vi "Actor Core.vi"(8 "error in":errorcluster, 11 "Test Node View in":refnum<class "Test Node View.lvclass">) -> (0 "error out":errorcluster, 3 "Actor out":refnum<class "Actor.lvclass">)   [LabVIEW 2013, in "Test Node View.lvlib" / "Test Node View.lvclass"]
doc: "(<B>Filename</B>: Actor Framework.lvlib:Actor.lvclass:Actor Core.vi)\n\nReceives messages to the actor, reacts to them, and initiates any error handling that may shut the actor down.\n\nDescendant classes may override this VI to append parallel tasks for the actor to complete while it handles messages. Overrides use the Call Parent Method node."
uses:
  Test Node View.lvclass
  <vilib>/ActorFramework/Actor/Actor.lvclass
  Resources/UI Controls/Tiles.ctl
  Resources/UI Controls/Tile.ctl
  Resources/UI Controls/Add Tile.ctl
  Resources/UI Controls/Delete Frame.ctl
  Test Node View.lvclass/Test Node View.ctl
  <vilib>/ActorFramework/Actor/Actor.lvclass/Actor.ctl
  <vilib>/ActorFrameworkMVC/View Actor/View Actor.lvclass
  <vilib>/ActorFramework/Message Enqueuer/Message Enqueuer.lvclass/Message Enqueuer.ctl
  Test Node View Messages/Set Frame Visibility Msg/Set Frame Visibility Msg.lvclass/Set Frame Visibility Msg.ctl
  Test Node View Messages/Update Tiles Msg/Update Tiles Msg.lvclass/Update Tiles Msg.ctl
  <vilib>/ActorFrameworkMVC/UI Controller Messages/Move Splitter Msg/Move Splitter Msg.lvclass/Move Splitter Msg.ctl
  <vilib>/Utility/miscctls.llb/LVPositionTypeDef.ctl
  <vilib>/ActorFrameworkMVC/UI Controller Messages/Move Subpanel Msg/Move Subpanel Msg.lvclass/Move Subpanel Msg.ctl
  <vilib>/ActorFrameworkMVC/UI Controller Messages/Insert Subpanel Msg/Insert Subpanel Msg.lvclass/Insert Subpanel Msg.ctl
  Models/Edit Test Node Model Messages/Set Framed Test Node Path Msg/Set Framed Test Node Path Msg.lvclass/Set Framed Test Node Path Msg.ctl
  Test Node View Messages/Move Frame Msg/Move Frame Msg.lvclass/Move Frame Msg.ctl
  Models/Test Node Model Messages/Set Framed Test Node Path Msg/Set Framed Test Node Path Msg.lvclass/Set Framed Test Node Path Msg.ctl
  Models/Test Channel Model Messages/Set Test Node Path Msg/Set Test Node Path Msg.lvclass/Set Test Node Path Msg.ctl
  <vilib>/ActorFramework/Message Enqueuer/Init from Existing Queue.vi
  <vilib>/ActorFramework/Message Enqueuer/Enqueue.vi
  <vilib>/ActorFramework/Message Priority Queue/Priority Enqueue.vi
  <vilib>/ActorFramework/Message Enqueuer/Message Enqueuer.lvclass
  Test Node View Messages/Set Frame Visibility Msg/Set Frame Visibility Msg.lvclass
  Test Node View Messages/Update Tiles Msg/Update Tiles Msg.lvclass
  Test Node View Messages/Move In Previous Page Msg/Move In Previous Page Msg.lvclass
  Test Node View Messages/Move In Next Page Msg/Move In Next Page Msg.lvclass
  <vilib>/ActorFrameworkMVC/UI Controller Messages/Move Splitter Msg/Move Splitter Msg.lvclass
  <vilib>/ActorFrameworkMVC/UI Controller Messages/Move Subpanel Msg/Move Subpanel Msg.lvclass
  <vilib>/ActorFrameworkMVC/UI Controller Messages/Insert Subpanel Msg/Insert Subpanel Msg.lvclass
  Models/Project Model Messages/Preview Project Msg/Preview Project Msg.lvclass
  Models/Project Model Messages/Update Tiles Info Msg/Update Tiles Info Msg.lvclass
  Models/Project Model Messages/Update Previous Button Visibility Msg/Update Previous Button Visibility Msg.lvclass
  Models/Project Model Messages/Update Next Button Visibility Msg/Update Next Button Visibility Msg.lvclass
  Models/Create Test Node Model Messages/Reinitialize All Msg/Reinitialize All Msg.lvclass
  Models/Create Test Node Model Messages/Key Focus Msg/Key Focus Msg.lvclass
  Test Node View Messages/Move Out Next Page Msg/Move Out Next Page Msg.lvclass
  Models/Test Node Model Messages/Next Page Msg/Next Page Msg.lvclass
  Test Node View Messages/Move Out Previous Page Msg/Move Out Previous Page Msg.lvclass
  Models/Test Node Model Messages/Previous Page Msg/Previous Page Msg.lvclass
  Models/Edit Test Node Model Messages/Set Framed Test Node Path Msg/Set Framed Test Node Path Msg.lvclass
  Models/Edit Test Node Model Messages/Initialize Edit Test Node Msg/Initialize Edit Test Node Msg.lvclass
  Test Node View Messages/Move Frame Msg/Move Frame Msg.lvclass
  Models/Test Node Model Messages/Set Framed Test Node Path Msg/Set Framed Test Node Path Msg.lvclass
  Models/Test Channel Model Messages/Set Test Node Path Msg/Set Test Node Path Msg.lvclass
  <vilib>/ActorFrameworkMVC/View Actor Messages/Get Model Enqueuer Msg/Get Model Enqueuer Msg.lvclass
  <vilib>/ActorFrameworkMVC/UI Controller Messages/Get Model Actor Enqueuer Msg/Get Model Actor Enqueuer Msg.lvclass
panel:
  in  "Frame":T1
  in  "Previous Button":bool
  in  "Next Button":bool
  in  "Add Tile":T2
  out "Tiles":T3
  in  "Back":bool
  # "测试节点"
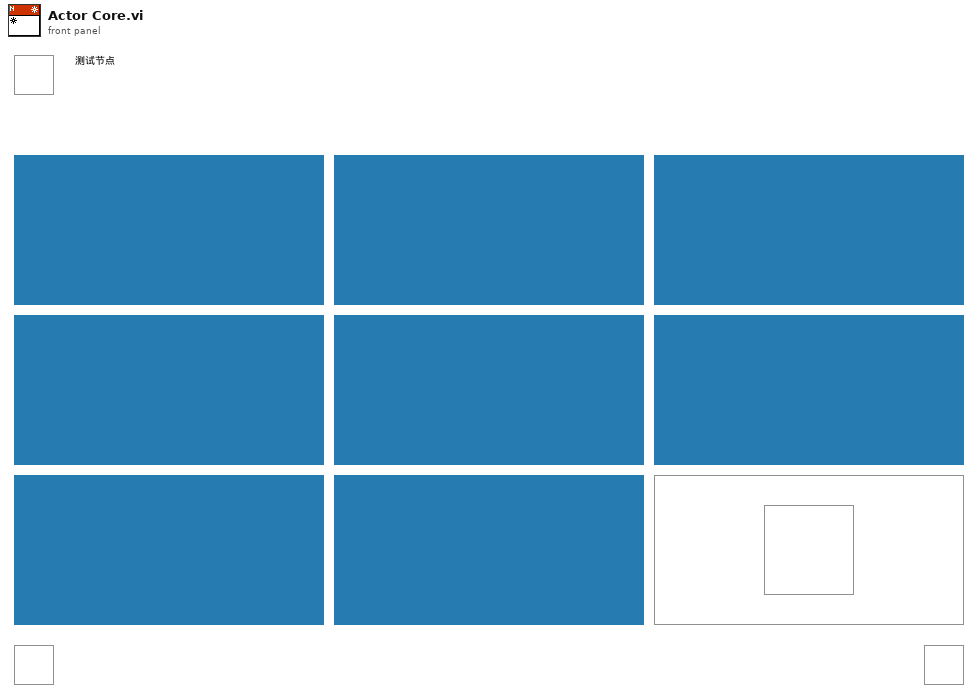
[diagram p1: front panel]
types:
  T1 = typedef "Delete Frame.ctl" = bool
  T2 = typedef "Add Tile.ctl" = bool
  T3 = typedef "Tiles.ctl" = cluster{"Tile 1":T4, "Tile 2":T4, "Tile 3":T4, "Tile 4":T4, "Tile 5":T4, "Tile 6":T4, "Tile 7":T4, "Tile 8":T4}
  T4 = typedef "Tile.ctl" = cluster{"Name":string, "Spec":string, "File Path":string}
  T5 = typedef "Test Node View.lvlib/Test Node View.lvclass/Events.ctl" = cluster{"Update Tiles Info":refnum<user-event>, "Set Previous Button Visibility":refnum<user-event>, "Set Next Button Visibility":refnum<user-event>, "Move In Previous":refnum<user-event>, "Move In Next":refnum<user-event>}
  T6 = typedef "LVPositionTypeDef.ctl" = cluster{"Left":i32, "Top":i32}
  T7 = enum8{"Enabled", "Disabled", "Disabled and Grayed Out"}
  T8 = typedef "Info Cluster.ctl" = cluster{"Name":string, "Spec":string, "File Path":string}
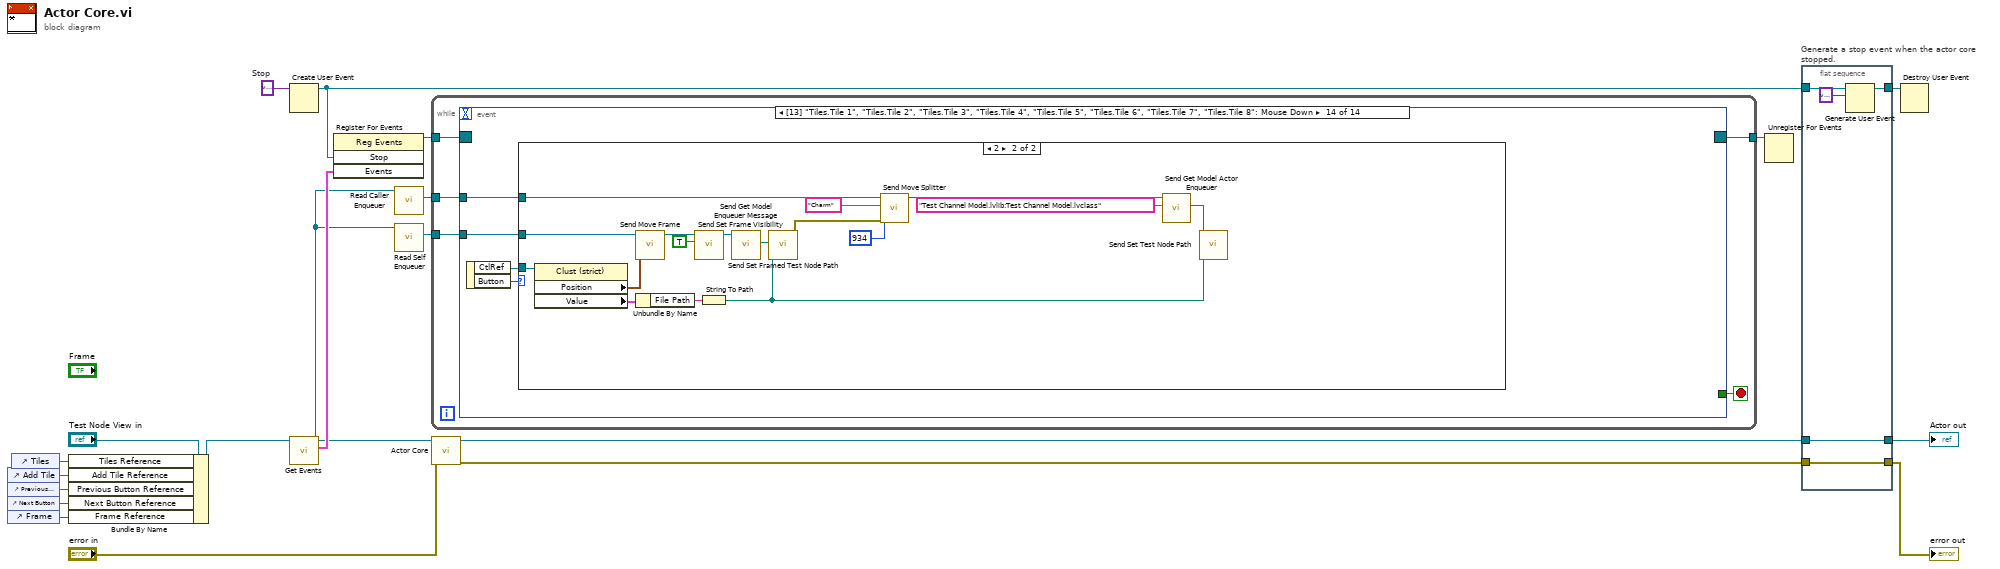
[diagram p0: block diagram]
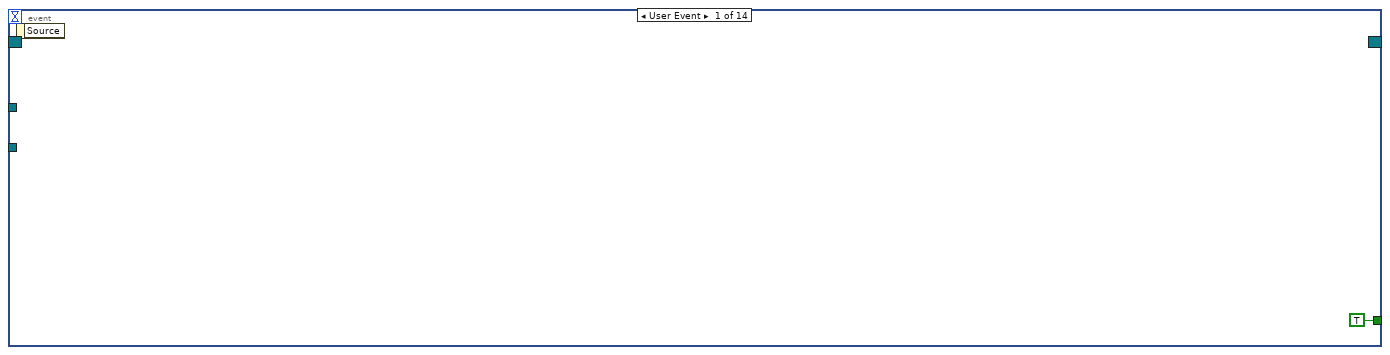
[diagram p2: hidden frame]
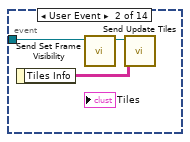
[diagram p3: hidden frame]
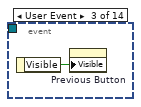
[diagram p4: hidden frame]
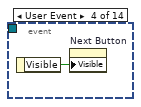
[diagram p5: hidden frame]
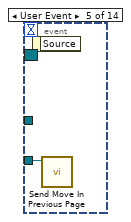
[diagram p6: hidden frame]
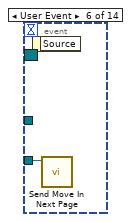
[diagram p7: hidden frame]
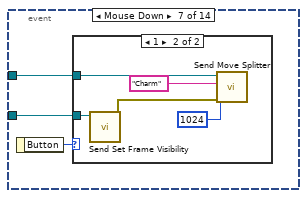
[diagram p8: hidden frame]
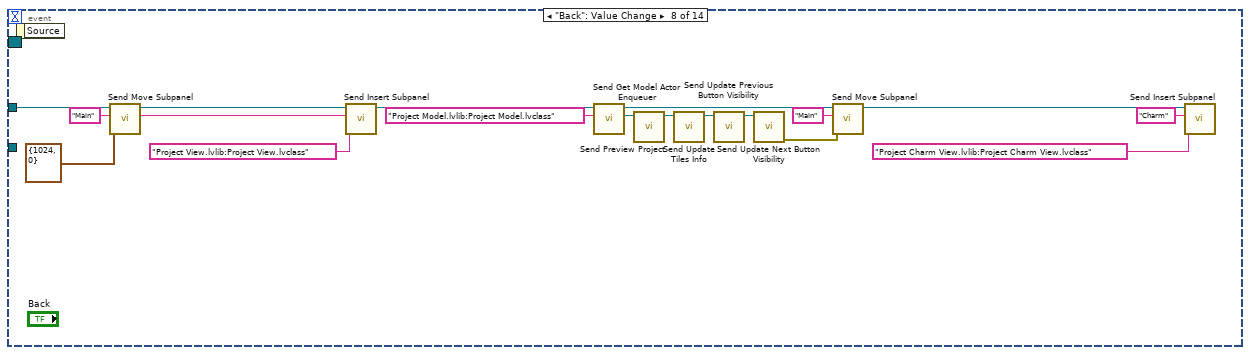
[diagram p10: hidden frame]
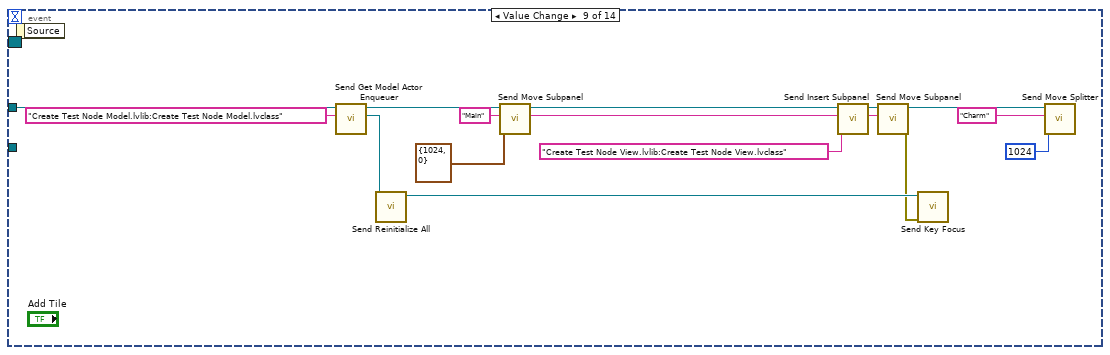
[diagram p11: hidden frame]
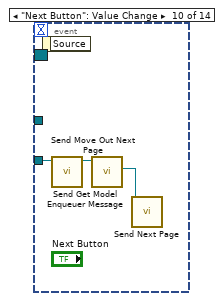
[diagram p12: hidden frame]
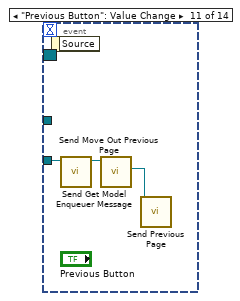
[diagram p13: hidden frame]
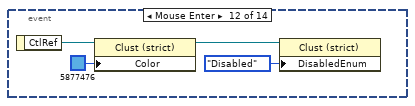
[diagram p14: hidden frame]
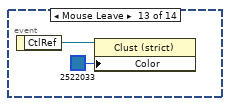
[diagram p15: hidden frame]
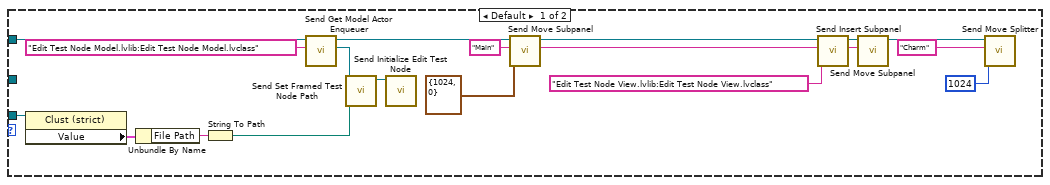
[diagram p16: hidden frame]
diagram:
  w21 = variant  # Stop
  n1 = control-ref of="Add Tile"() -> (w4:refnum<vi>)
  n2 = control-ref of="Previous Button"() -> (w5:refnum<vi>)
  n3 = control-ref of="Next Button"() -> (w6:refnum<vi>)
  n4 = control-ref of="Frame"() -> (w7:refnum<vi>)
  n5 = control-ref of="Tiles"() -> (w8:refnum<vi>)
  n6 = Bundle By Name(cluster="Test Node View in", "Tiles Reference"=w8, "Add Tile Reference"=w4, "Previous Button Reference"=w5, "Next Button Reference"=w6, "Frame Reference"=w7) -> (w9:refnum<class "Test Node View.lvclass">)
  n7 = Create User Event(user event datatype=w21) -> (user event=w12:refnum<user-event>)  [unwired: 1 in, 1 out]
  n8 = call "Get Events.vi"("Test Node View in"=w9) -> ("Events"=w11:T5, "Test Node View out"=w3:refnum<class "Test Node View.lvclass">)  [unwired: 9 in]
  n9 = register-events(w12, w11) -> (reference out=w13:refnum<event-registration>)  [unwired: 2 in, 1 out]
  n10 = call <vilib>:"Read Caller Enqueuer.vi"("Actor"=w3) -> ("Caller Enqueuer"=w2:refnum<class "Message Enqueuer.lvclass">)  [unwired: 10 in]
  n11 = call <vilib>:"Read Self Enqueuer.vi"("Actor"=w3) -> ("Self Enqueuer"=w1:refnum<class "Message Enqueuer.lvclass">)  [unwired: 10 in]
  n12 = while {
    tunnel: [w26] -> w10
    tunnel: w13 -> [w24]
    tunnel: w2 -> [w23]
    tunnel: w1 -> [w22]
    stop <- w25 stop-if-true
    n13 = event shown="[13] \"Tiles.Tile 1\", \"Tiles.Tile 2\", \"Tiles.Tile 3\", \"Tiles.Tile 4\", \"Tiles.Tile 5\", \"Tiles.Tile 6\", \"Tiles.Tile 7\", \"Tiles.Tile 8\": Mouse Down" {
      selector: w24 -> [_ _ _ _ _ _ _ _ _ _ _ _ _ _]
      dyn-events: [_ _ _ _ _ _ _ _ _ _ _ _ _ _] -> w26
      timeout: _ -> [_ _ _ _ _ _ _ _ _ _ _ _ _ _]
      tunnel: [TRUE _ _ _ _ _ _ _ _ _ _ _ _ _] -> w25
      tunnel: w23 -> [_ _ _ _ _ _ w37 w43 w73 _ _ _ _ w86]
      tunnel: w22 -> [_ w30 _ _ w33 w34 w35 _ _ w75 w78 _ _ w87]
      event User Event {
        n14 = event-data() -> ()  [unwired: 1 in, 1 out]
      }
      event User Event {
        n15 = event-data() -> ("Tiles Info"=w28:string[][])  [unwired: 1 in]
        n16 = call "Send Set Frame Visibility.vi"("Message Enqueuer"=w30) -> ("Message Enqueuer out"=w29:refnum<class "Message Enqueuer.lvclass">)  [unwired: 9 in, 1 out]
        n17 = call "Send Update Tiles.vi"("Sensor Tiles Info"=w28, "Message Enqueuer"=w29) -> ()  [unwired: 8 in, 2 out]
      }
      event User Event {
        n18 = event-data() -> ("Visible"=w31:bool)  [unwired: 1 in]
        n19 = property on="Previous Button" class="Bool"("Visible"=w31) -> ()  [unwired: 2 in, 2 out]
      }
      event User Event {
        n20 = event-data() -> ("Visible"=w32:bool)  [unwired: 1 in]
        n21 = property on="Next Button" class="Bool"("Visible"=w32) -> ()  [unwired: 2 in, 2 out]
      }
      event User Event {
        n22 = event-data() -> ()  [unwired: 1 in, 1 out]
        n23 = call "Send Move In Previous Page.vi"("Message Enqueuer"=w33) -> ()  [unwired: 9 in, 2 out]
      }
      event User Event {
        n24 = event-data() -> ()  [unwired: 1 in, 1 out]
        n25 = call "Send Move In Next Page.vi"("Message Enqueuer"=w34) -> ()  [unwired: 9 in, 2 out]
      }
      event Mouse Down {
        n26 = event-data() -> ("Button"=w36:u16)  [unwired: 1 in]
        n27 = case shown="1" w36 {
          tunnel: w37 -> [_ w42]
          tunnel: w35 -> [_ w39]
          frame 0, Default {
          }
          frame 1 {
            n28 = call "Send Set Frame Visibility.vi"("Message Enqueuer"=w39) -> ("error out"=w38:errorcluster)  [unwired: 9 in, 1 out]
            n29 = call <vilib>:"Send Move Splitter.vi"("error in (no error)"=w38, "Splitter Position"=1024, "Splitter Name"="Charm", "Message Enqueuer"=w42) -> ()  [unwired: 6 in, 2 out]
          }
        }
      }
      event "Back": Value Change {
        w56 = "Main" ("Subpanel Name")
        n30 = event-data() -> ()  [unwired: 1 in, 1 out]
        n31 = call <vilib>:"Send Move Subpanel.vi"("Position (0,0)"=T6 {"Left"=1024, "Top"=0}, "Subpanel Name"=w56, "Message Enqueuer"=w43) -> ("Message Enqueuer out"=w59:refnum<class "Message Enqueuer.lvclass">)  [unwired: 7 in, 1 out]
        n32 = call <vilib>:"Send Insert Subpanel.vi"("View Name"="Project View.lvlib:Project View.lvclass" ("Subpanel Name"), "Subpanel Name"=w56, "Message Enqueuer"=w59) -> ("Message Enqueuer out"=w53:refnum<class "Message Enqueuer.lvclass">)  [unwired: 7 in, 1 out]
        n33 = call <vilib>:"Send Get Model Actor Enqueuer.vi"("Model Name"="Project Model.lvlib:Project Model.lvclass", "Message Enqueuer in"=w53) -> ("Reply"=w44:refnum<class "Message Enqueuer.lvclass">, "Message Enqueuer out"=w52:refnum<class "Message Enqueuer.lvclass">)  [unwired: 6 in, 2 out]
        n34 = call "Send Preview Project.vi"("Message Enqueuer"=w44) -> ("Message Enqueuer out"=w54:refnum<class "Message Enqueuer.lvclass">)  [unwired: 9 in, 1 out]
        n35 = call "Send Update Tiles Info.vi"("Message Enqueuer"=w54) -> ("Message Enqueuer out"=w50:refnum<class "Message Enqueuer.lvclass">)  [unwired: 9 in, 1 out]
        n36 = call "Send Update Previous Button Visibility.vi"("Message Enqueuer"=w50) -> ("Message Enqueuer out"=w49:refnum<class "Message Enqueuer.lvclass">)  [unwired: 9 in, 1 out]
        n37 = call "Send Update Next Button Visibility.vi"("Message Enqueuer"=w49) -> ("error out"=w48:errorcluster)  [unwired: 9 in, 1 out]
        n38 = call <vilib>:"Send Move Subpanel.vi"("error in (no error)"=w48, "Subpanel Name"="Main", "Message Enqueuer"=w52) -> ("Message Enqueuer out"=w47:refnum<class "Message Enqueuer.lvclass">)  [unwired: 7 in, 1 out]
        n39 = call <vilib>:"Send Insert Subpanel.vi"("View Name"="Project Charm View.lvlib:Project Charm View.lvclass", "Subpanel Name"="Charm", "Message Enqueuer"=w47) -> ()  [unwired: 7 in, 2 out]
      }
      event Value Change {
        w69 = "Main" ("Subpanel Name")
        n40 = event-data() -> ()  [unwired: 1 in, 1 out]
        n41 = call <vilib>:"Send Get Model Actor Enqueuer.vi"("Model Name"="Create Test Node Model.lvlib:Create Test Node Model.lvclass", "Message Enqueuer in"=w73) -> ("Reply"=w62:refnum<class "Message Enqueuer.lvclass">, "Message Enqueuer out"=w63:refnum<class "Message Enqueuer.lvclass">)  [unwired: 6 in, 2 out]
        n42 = call "Send Reinitialize All.vi"("Message Enqueuer"=w62) -> ("Message Enqueuer out"=w61:refnum<class "Message Enqueuer.lvclass">)  [unwired: 9 in, 1 out]
        n43 = call <vilib>:"Send Move Subpanel.vi"("Position (0,0)"=T6 {"Left"=1024, "Top"=0}, "Subpanel Name"=w69, "Message Enqueuer"=w63) -> ("Message Enqueuer out"=w72:refnum<class "Message Enqueuer.lvclass">)  [unwired: 7 in, 1 out]
        n44 = call <vilib>:"Send Insert Subpanel.vi"("View Name"="Create Test Node View.lvlib:Create Test Node View.lvclass", "Subpanel Name"=w69, "Message Enqueuer"=w72) -> ("Message Enqueuer out"=w70:refnum<class "Message Enqueuer.lvclass">)  [unwired: 7 in, 1 out]
        n45 = call <vilib>:"Send Move Subpanel.vi"("Subpanel Name"=w69, "Message Enqueuer"=w70) -> ("error out"=w60:errorcluster, "Message Enqueuer out"=w68:refnum<class "Message Enqueuer.lvclass">)  [unwired: 8 in]
        n46 = call "Send Key Focus.vi"("error in (no error)"=w60, "Message Enqueuer"=w61) -> ()  [unwired: 8 in, 2 out]
        n47 = call <vilib>:"Send Move Splitter.vi"("Splitter Position"=1024, "Splitter Name"="Charm", "Message Enqueuer"=w68) -> ()  [unwired: 7 in, 2 out]
      }
      event "Next Button": Value Change {
        n48 = event-data() -> ()  [unwired: 1 in, 1 out]
        n49 = call "Send Move Out Next Page.vi"("Message Enqueuer"=w75) -> ("Message Enqueuer out"=w74:refnum<class "Message Enqueuer.lvclass">)  [unwired: 9 in, 1 out]
        n50 = call <vilib>:"Send Get Model Enqueuer Message.vi"("Message Enqueuer in"=w74) -> ("Reply"=w76:refnum<class "Message Enqueuer.lvclass">)  [unwired: 7 in, 3 out]
        n51 = call "Send Next Page.vi"("Message Enqueuer"=w76) -> ()  [unwired: 9 in, 2 out]
      }
      event "Previous Button": Value Change {
        n52 = event-data() -> ()  [unwired: 1 in, 1 out]
        n53 = call "Send Move Out Previous Page.vi"("Message Enqueuer"=w78) -> ("Message Enqueuer out"=w77:refnum<class "Message Enqueuer.lvclass">)  [unwired: 9 in, 1 out]
        n54 = call <vilib>:"Send Get Model Enqueuer Message.vi"("Message Enqueuer in"=w77) -> ("Reply"=w79:refnum<class "Message Enqueuer.lvclass">)  [unwired: 7 in, 3 out]
        n55 = call "Send Previous Page.vi"("Message Enqueuer"=w79) -> ()  [unwired: 9 in, 2 out]
      }
      event Mouse Enter {
        n56 = event-data() -> ("CtlRef"=w80:refnum<vi>)  [unwired: 1 in]
        n57 = property class="Clust (strict)"(reference=w80, "Color"=u32 5877476) -> (reference out=w82:refnum<vi>)  [unwired: 1 in, 1 out]
        n58 = property class="Clust (strict)"(reference=w82, "DisabledEnum"=T7."Disabled" ("Disabled")) -> ()  [unwired: 1 in, 2 out]
      }
      event Mouse Leave {
        n59 = event-data() -> ("CtlRef"=w84:refnum<vi>)  [unwired: 1 in]
        n60 = property class="Clust (strict)"(reference=w84, "Color"=u32 2522033) -> ()  [unwired: 1 in, 2 out]
      }
      event Mouse Down {
        n61 = event-data() -> ("CtlRef"=w89:refnum<vi>, "Button"=w88:u16)  [unwired: 1 in]
        n62 = case shown="2" w88 {
          tunnel: w89 -> [w105 w123]
          tunnel: w87 -> [_ w122]
          tunnel: w86 -> [w106 w118]
          frame Default {
            w94 = "Main" ("Subpanel Name")
            n63 = property class="Clust (strict)"(reference=w105) -> ("Value"=w102:T4)  [unwired: 1 in, 2 out]
            n64 = Unbundle By Name(w102) -> ("File Path"=w101:string)
            n65 = String To Path(string=w101) -> (path=w100:path)
            n66 = call <vilib>:"Send Get Model Actor Enqueuer.vi"("Model Name"="Edit Test Node Model.lvlib:Edit Test Node Model.lvclass", "Message Enqueuer in"=w106) -> ("Reply"=w103:refnum<class "Message Enqueuer.lvclass">, "Message Enqueuer out"=w90:refnum<class "Message Enqueuer.lvclass">)  [unwired: 6 in, 2 out]
            n67 = call "Send Set Framed Test Node Path.vi"("Framed Test Node Path"=w100, "Message Enqueuer"=w103) -> ("Message Enqueuer out"=w99:refnum<class "Message Enqueuer.lvclass">)  [unwired: 8 in, 1 out]
            n68 = call "Send Initialize Edit Test Node.vi"("Message Enqueuer"=w99) -> ()  [unwired: 9 in, 2 out]
            n69 = call <vilib>:"Send Move Subpanel.vi"("Position (0,0)"=T6 {"Left"=1024, "Top"=0}, "Subpanel Name"=w94, "Message Enqueuer"=w90) -> ("Message Enqueuer out"=w91:refnum<class "Message Enqueuer.lvclass">)  [unwired: 7 in, 1 out]
            n70 = call <vilib>:"Send Insert Subpanel.vi"("View Name"="Edit Test Node View.lvlib:Edit Test Node View.lvclass", "Subpanel Name"=w94, "Message Enqueuer"=w91) -> ("Message Enqueuer out"=w93:refnum<class "Message Enqueuer.lvclass">)  [unwired: 7 in, 1 out]
            n71 = call <vilib>:"Send Move Subpanel.vi"("Subpanel Name"=w94, "Message Enqueuer"=w93) -> ("Message Enqueuer out"=w95:refnum<class "Message Enqueuer.lvclass">)  [unwired: 8 in, 1 out]
            n72 = call <vilib>:"Send Move Splitter.vi"("Splitter Position"=1024, "Splitter Name"="Charm", "Message Enqueuer"=w95) -> ()  [unwired: 7 in, 2 out]
          }
          frame 2 {
            n73 = property class="Clust (strict)"(reference=w123) -> ("Position"=w121:T6, "Value"=w114:T8)  [unwired: 1 in, 2 out]
            n74 = call "Send Move Frame.vi"("Position"=w121, "Message Enqueuer"=w122) -> ("Message Enqueuer out"=w120:refnum<class "Message Enqueuer.lvclass">)  [unwired: 8 in, 1 out]
            n75 = Unbundle By Name(w114) -> ("File Path"=w113:string)
            n76 = call "Send Set Frame Visibility.vi"("Visible (F)"=TRUE, "Message Enqueuer"=w120) -> ("Message Enqueuer out"=w115:refnum<class "Message Enqueuer.lvclass">)  [unwired: 8 in, 1 out]
            n77 = String To Path(string=w113) -> (path=w107:path)
            n78 = call <vilib>:"Send Get Model Enqueuer Message.vi"("Message Enqueuer in"=w115) -> ("Reply"=w111:refnum<class "Message Enqueuer.lvclass">)  [unwired: 7 in, 3 out]
            n79 = call "Send Set Framed Test Node Path.vi"("Framed Test Node Path"=w107, "Message Enqueuer"=w111) -> ("error out"=w112:errorcluster)  [unwired: 8 in, 1 out]
            n80 = call <vilib>:"Send Move Splitter.vi"("error in (no error)"=w112, "Splitter Position"=934, "Splitter Name"="Charm", "Message Enqueuer"=w118) -> ("Message Enqueuer out"=w110:refnum<class "Message Enqueuer.lvclass">)  [unwired: 6 in, 1 out]
            n81 = call <vilib>:"Send Get Model Actor Enqueuer.vi"("Model Name"="Test Channel Model.lvlib:Test Channel Model.lvclass", "Message Enqueuer in"=w110) -> ("Reply"=w108:refnum<class "Message Enqueuer.lvclass">)  [unwired: 6 in, 3 out]
            n82 = call "Send Set Test Node Path.vi"("Test Node Path"=w107, "Message Enqueuer"=w108) -> ()  [unwired: 8 in, 2 out]
          }
        }
      }
    }
  }
  n83 = call-parent "Actor Core.vi"("error in"="error in", "View Actor in"=w3) -> ("error out"=w16:errorcluster, "Actor out"=w17:refnum<class "Actor.lvclass">)  [unwired: 8 in]
  n84 = Unregister For Events(event registration refnum=w10) -> ()  [unwired: 1 in, 1 out]
  n85 = flat-sequence "Generate a stop event when the actor core stopped." {
    tunnel: w12 -> [w128]
    tunnel: [w126] -> w20
    tunnel: w17 -> [w125]
    tunnel: w16 -> [w124]
    tunnel: [w125] -> w15
    tunnel: [w124] -> w14
    frame #0 {
      n86 = Generate User Event(user event=w128, event data cluster=variant ("event data")) -> (user event out=w126:refnum<user-event>)  [unwired: 2 in, 1 out]
    }
  }
  n87 = Destroy User Event(user event=w20) -> ()  [unwired: 1 in, 1 out]
  "error out" <- w14
  "Actor out" <- w15
